vi "Fit Transform.vi"(8 "error in (no error)":errorcluster caption="entrée d'erreur (pas d'erreur)", 9 "y":string[][](array[string]), 10 "X":string[][](array[string]), 11 "IterativeImputer.lvclass":refnum<class "IterativeImputer.lvclass">) -> (0 "error out":errorcluster caption="sortie d'erreur", 2 "Data":T1, 3 "IterativeImputer.lvclass":refnum<class "IterativeImputer.lvclass">)   [LabVIEW 2020, in "IterativeImputer.lvclass"]
doc: "Fits the imputer on X and return the transformed X.\n\nReturns : \n\n- Xt : array-like, shape (n_samples, n_features)\nThe imputed input data."
uses:
  IterativeImputer.lvclass
  IterativeImputer.lvclass/IterativeImputer.ctl
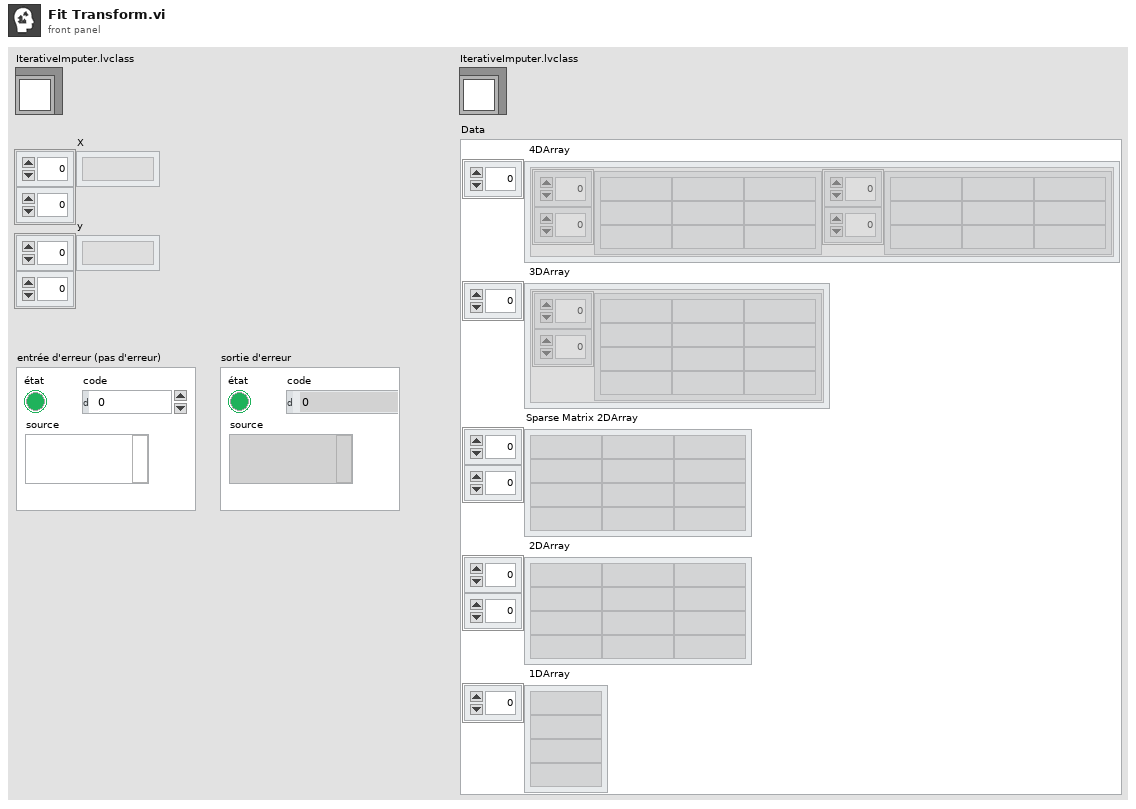
[diagram p1: front panel]
types:
  T1 = cluster{" 4DArray":cluster{"1":string[][], "2":string[][]}[], " 3DArray":cluster{"Tableau":string[][]}[], "Sparse Matrix 2DArray":string[][], " 2DArray":string[][], " 1DArray":string[]}
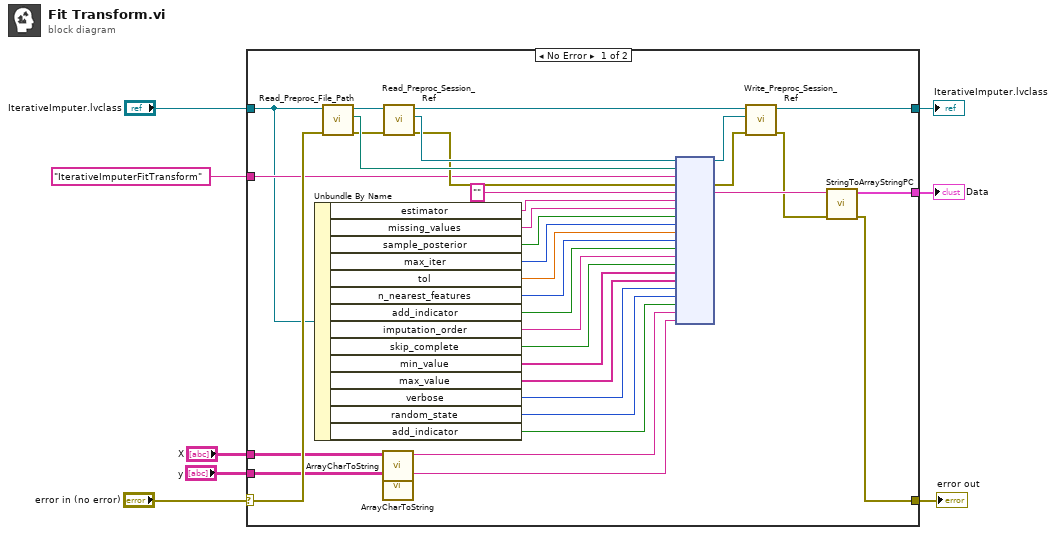
[diagram p0: block diagram]
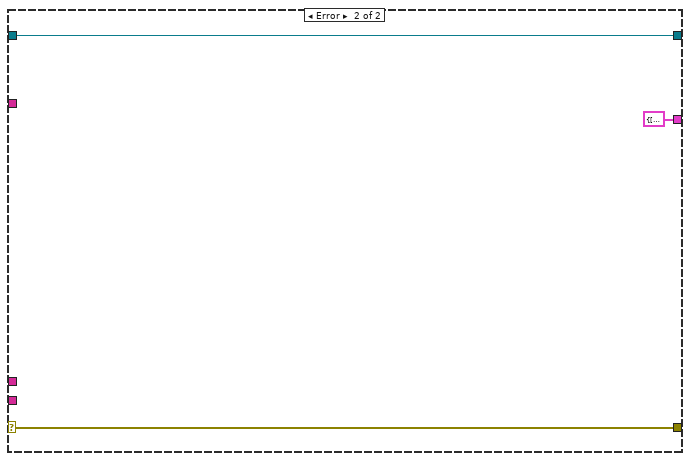
[diagram p2: hidden frame]
diagram:
  n1 = case shown="No Error" "error in (no error)" {
    selector: "error in (no error)" -> [w34 w46]
    tunnel: [w14 w46] -> w7
    tunnel: [w17 w45] -> w5
    tunnel: "IterativeImputer.lvclass" -> [w32 w45]
    tunnel: "IterativeImputerFitTransform" ("Fonction") -> [w33 _]
    tunnel: "X" -> [w12 _]
    tunnel: "y" -> [w10 _]
    tunnel: [w13 T1 {" 4DArray"=[], " 3DArray"=[], "Sparse Matrix 2DArray"=[], " 2DArray"=[], " 1DArray"=[]} ("Data")] -> w1
    frame No Error {
      n2 = Unbundle By Name(w32) -> ("estimator"=w31:string, "missing_values"=w30:string, "sample_posterior"=w29:bool, "max_iter"=w28:i32, "tol"=w27:dbl, "n_nearest_features"=w26:i32, "add_indicator"=w25:bool, "imputation_order"=w24:string, "skip_complete"=w23:bool, "min_value"=w22:string[], "max_value"=w21:string[], "verbose"=w20:i32, "random_state"=w19:i32, "add_indicator"=w18:bool)
      n3 = call-dynamic "Read_Preproc_File_Path.vi"("error in (no error)"=w34, "Python in"=w32) -> ("error out"=w38:errorcluster, "File_Path"=w41:path, "Python out"=w43:refnum<class "IterativeImputer.lvclass">)  [unwired: 7 in]
      n4 = call "ArrayCharToString.vi"("TAB"=w12) -> ("Instruction"=w11:string)  [unwired: 10 in]
      n5 = call "ArrayCharToString.vi"("TAB"=w10) -> ("Instruction"=w9:string)  [unwired: 10 in]
      n6 = call-dynamic "Read_Preproc_Session_Ref.vi"("error in (no error)"=w38, "Python in"=w43) -> ("error out"=w39:errorcluster, "Session_ref"=w40:refnum<k35>, "Python out"=w42:refnum<class "IterativeImputer.lvclass">)  [unwired: 7 in]
      n7 = node(w40, w41, w33, w39, "", w31, w30, w29, w28, w27, w26, w25, w24, w23, w22, w21, w20, w19, w18, w11, w9) -> (w35:refnum<k35>, w37:errorcluster, w16:string)  [unwired: 16 in, 2 out]
      n8 = call-dynamic "Write_Preproc_Session_Ref.vi"("error in (no error)"=w37, "Session_ref"=w35, "Python in"=w42) -> ("error out"=w15:errorcluster, "Python out"=w17:refnum<class "IterativeImputer.lvclass">)  [unwired: 7 in]
      n9 = call "StringToArrayStringPC.vi"("sortie d'erreur"=w15, "Return value"=w16) -> ("sortie d'erreur"=w14:errorcluster, "Data"=w13:T1)  [unwired: 8 in]
    }
    frame Error {
    }
  }
  "error out" <- w7
  "IterativeImputer.lvclass" <- w5
  "Data" <- w1
